vi "Basic Read Sensor Data.vi"() -> ()   [LabVIEW 2017]
doc: "Purpose: Quick example to retrieve the data from the sensor channel\nHardware setup: At least one Fluigent sensor"
uses:
  TypeDefs/fgt_CHANNEL_INFO.ctl
  TypeDefs/fgt_INSTRUMENT_TYPE.ctl
  TypeDefs/fgt_SENSOR_UNIT.ctl
  fgt_SDK.lvlib
panel:
  out "Sensor(s)":T4(array[cluster]) {"fgt_CHANNEL_INFO"."indexID" format="%.0x"; "fgt_CHANNEL_INFO"."index" format="%.0x"; "fgt_CHANNEL_INFO"."position" format="%.0x"; "fgt_CHANNEL_INFO"."DeviceSN" format="%.0x"; "fgt_CHANNEL_INFO"."firmware" format="%.0x"; "fgt_CHANNEL_INFO"."ControllerSN" format="%.0x"}
  out "error out":errorcluster
  # "Hit the \"Run\" button to retrieve information about all Fluigent connected sensors"
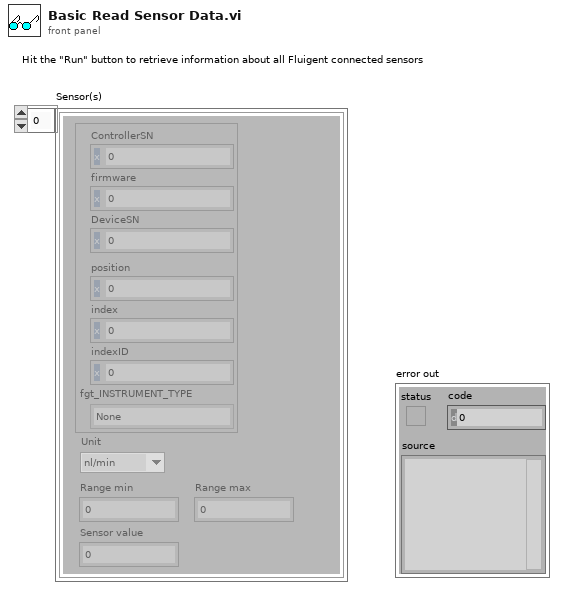
[diagram p1: front panel]
types:
  T1 = typedef "fgt_SDK.lvlib/fgt_CHANNEL_INFO.ctl" = cluster{"ControllerSN":u16, "firmware":u16, "DeviceSN":u16, "position":u32, "index":u32, "indexID":u32, "fgt_INSTRUMENT_TYPE":T2}
  T2 = typedef "fgt_SDK.lvlib/fgt_INSTRUMENT_TYPE.ctl" = enum32{"None", "MFCS", "MFCS_EZ", "FRP", "LineUP", "IPS"}
  T3 = typedef "fgt_SDK.lvlib/fgt_SENSOR_UNIT.ctl" = enum16{"nl/min", "µl/s", "µl/min", "ul/h", "ml/min", "ml/h", "mbar", "PSI", "bar"}
  T4 = cluster{"fgt_CHANNEL_INFO":T1, "Range min":dbl, "Range max":dbl, "Sensor value":dbl, "Unit":T3}[]
  T5 = cluster{"fgt_CHANNEL_INFO":T1, "Range min":dbl, "Range max":dbl, "Sensor value":dbl, "Unit":T3}
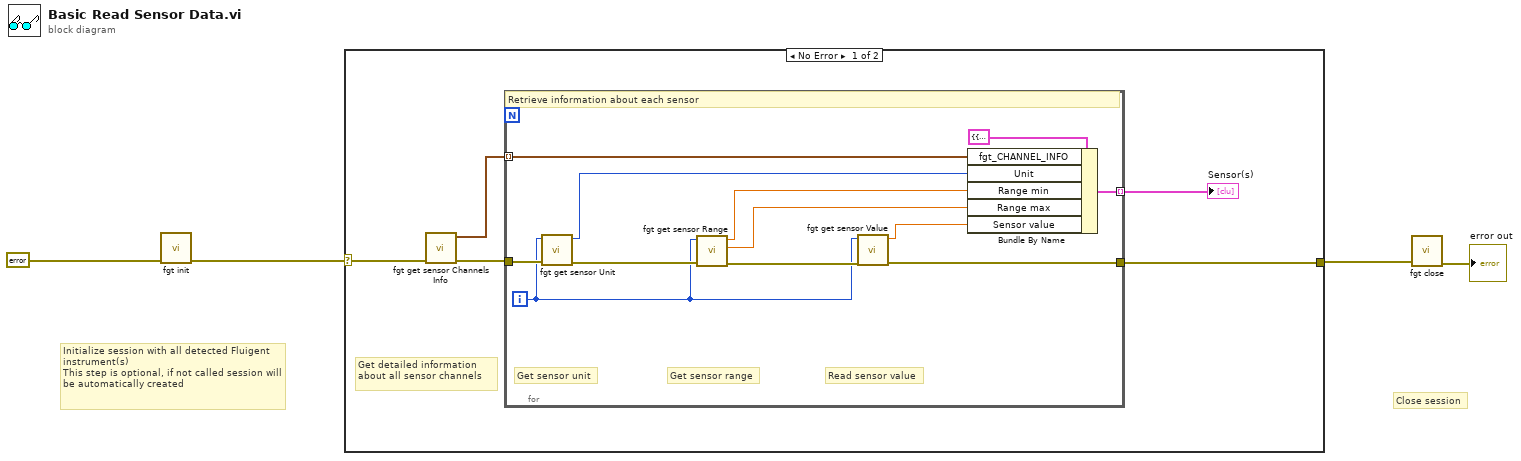
[diagram p0: block diagram]
diagram:
  # "Close session"
  # "Initialize session with all detected Fluigent instrument(s)\nThis step is optional, if not called session will be automatically created"
  n1 = call "fgt init.vi"("error in (no error)"=errorcluster {"status"=FALSE, "code"=0, "source"=""}) -> ("error out"=w2:errorcluster)  [unwired: 10 in]
  n2 = case shown="No Error" w2 {
    selector: w2 -> [w9 w22]
    tunnel: [w6 w22] -> w1
    frame No Error {
      # "Get detailed information about all sensor channels"
      n3 = call "fgt get sensor Channels Info.vi"("error in (no error)"=w9) -> ("error out"=w8:errorcluster, "Sensor channels info"=w7:T1[])  [unwired: 8 in, 1 out]
      n4 = for {
        tunnel: w8 -> [w21]
        tunnel: w7 -> [w17] mode=indexing
        tunnel: [w18] -> w6
        tunnel: [w15] -> w5 mode=indexing
        i -> [w10]
        # "Read sensor value"
        # "Get sensor range"
        # "Get sensor unit"
        # "Retrieve information about each sensor"
        n5 = call "fgt get sensor Unit.vi"("error in (no error)"=w21, "sensorIndex"=w10) -> ("error out"=w20:errorcluster, "unit out"=w14:T3)  [unwired: 8 in]
        n6 = call "fgt get sensor Range.vi"("error in (no error)"=w20, "sensorIndex"=w10) -> ("error out"=w19:errorcluster, "Smax out"=w12:sgl, "Smin out"=w13:sgl)  [unwired: 7 in]
        n7 = call "fgt get sensor Value.vi"("error in (no error)"=w19, "sensorIndex"=w10) -> ("error out"=w18:errorcluster, "value out"=w11:sgl)  [unwired: 8 in]
        n8 = Bundle By Name(cluster=T5 {"fgt_CHANNEL_INFO"={"ControllerSN"=0, "firmware"=0, "DeviceSN"=0, "position"=0, "index"=0, "indexID"=0, "fgt_INSTRUMENT_TYPE"=enum."None"}, "Range min"=0.0, "Range max"=0.0, "Sensor value"=0.0, "Unit"=enum."nl/min"} ("Cluster"), "fgt_CHANNEL_INFO"=w17, "Unit"=w14, "Range min"=w13, "Range max"=w12, "Sensor value"=w11) -> (w15:T5)
      }
      "Sensor(s)" <- w5
    }
    frame Error {
    }
  }
  n9 = call "fgt close.vi"("error in (no error)"=w1) -> ("error out"=→"error out":errorcluster)  [unwired: 10 in]
